vi "DMR_ImageRequestWaitFor.vi"(3 "queue number IN":i32, 4 "timeout(ms) IN":i32, 5 "driver handle IN":i32) -> (0 "error code OUT":i32, 1 "request number OUT":i32, 2 "driver handle OUT":i32)   [LabVIEW 2014]
doc: "Waits for an image request to become ready.\n\nThis function waits for an image request previously send to the camera by calling DMR_ImageRequestSingle.\n\nNote:\nWhenever a request is returned to the user the image data described by the request remains valid until the user unlocks the image buffer again or the device driver is closed.\n\nSee also:\nDMR_ImageRequestReset,\nDMR_ImageRequestSingle,\nDMR_ImageRequestUnlock,\nDMR_GetImageRequestInfo,\nDMR_GetImageRequestResult,\nDMR_GetImageRequestParamS\n\nThe 'error code OUT' terminal will deliver 0 if successful or a negative error code otherwise. A list of valid error codes and their meaning can be found in the manual about this interface."
uses:
  mvDeviceManager.dll
panel:
  # "OUTPUT"
  # "INPUT"
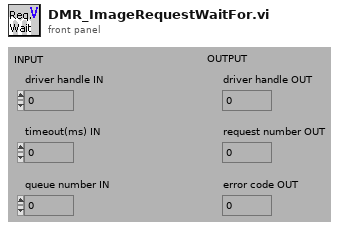
[diagram p1: front panel]
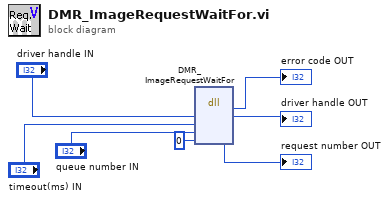
[diagram p0: block diagram]
diagram:
  n1 = dll-call lib="mvDeviceManager.dll" fn="DMR_ImageRequestWaitFor"("hDrv"="driver handle IN", "timeout_ms"="timeout(ms) IN", "queueNr"="queue number IN", "pRequestNr"=0 ("pRequestUsed")) -> (→"error code OUT":i32, "hDrv"=→"driver handle OUT":i32, "pRequestNr"=→"request number OUT":i32)  [unwired: 5 in, 2 out]
